vi "BRig_RT_panel_Laser2_v1,18.vi"(7 "input_setValues":bool, 9 "input_dataExp":u16[](array[numeric]), 11 "input_dataLC":u16[](array[numeric])) -> (1 "output_dataExp":u16[](array[numeric]), 3 "output_dataLC":u16[](array[numeric]))   [LabVIEW 2014]
panel:
  in  "LC_Wro_nRew2":u16
  in  "LC_Wro_nRew1":u16
  in  "LC_Rew_nRew2":u16
  in  "LC_Rew_nRew1":u16
  in  "LC_Sel_nRew2":u16
  in  "LC_Sel_nRew1":u16
  in  "LC_Cue_nRew2":u16
  in  "LC_Cue_nRew1":u16
  in  "LC_ENL_nRew2":u16
  in  "LC_ENL_nRew1":u16
  out "LaserPulseTrain":cluster{u16[], u16[]}(graph)
  in  "LED_baseline":bool
  in  "Laser_power_step":dbl
  in  "Laser_power_max":dbl
  in  "Laser_power_min":dbl
  in  "Laser_Tshutter":u16=2
  in  "Laser_Freq":u16=10
  in  "Laser_Tpeak":u16=2
  in  "Laser_T":u16
  in  "LC_Sel_PostR_Count":u16
  in  "LC_Sel_PostR_Probability":u16
  in  "LC_Sel_PostR_Block":u16(slide) max=2 step=1 scale=0.0..2.0
  in  "LC_Sel_PostR_OnOff":bool
  in  "LC_Sel_PostR_Tdelay":u16
  in  "LC_Cue_PostR_Count":u16
  in  "LC_Cue_PostR_delayOpt":bool
  in  "LC_Cue_PostR_Probability":u16
  in  "LC_Cue_PostR_Block":u16(slide) max=2 step=1 scale=0.0..2.0
  in  "LC_Cue_PostR_OnOff":bool
  in  "LC_Cue_PostR_Tdelay":u16
  in  "LC_ENL_PostR_delayOpt":bool
  in  "LC_ENL_PostR_Count":u16
  in  "LC_ENL_PostR_Probability":u16 max=100 step=1
  in  "LC_ENL_PostR_Block":u16(slide) max=2 step=1 scale=0.0..2.0
  in  "LC_ENL_PostR_OnOff":bool
  in  "LC_ENL_PostR_Tdelay":u16
  in  "LC_Sel_PreR_Count":u16
  in  "LC_Sel_First_Count":u16
  in  "LC_Sel_PreR_Probability":u16
  in  "LC_Sel_PreR_Block":u16(slide) max=2 step=1 scale=0.0..2.0
  in  "LC_Sel_PreR_OnOff":bool
  in  "LC_Sel_First_Probability":u16
  in  "LC_Sel_First_Block":u16(slide) max=2 step=1 scale=0.0..2.0
  in  "LC_Sel_First_OnOff":bool
  in  "LC_Sel_PreR_Tdelay":u16
  in  "LC_Sel_First_Tdelay":u16
  in  "LC_Cue_PreR_Count":u16
  in  "LC_Cue_First_Count":u16
  in  "LC_Cue_PreR_delayOpt":bool
  in  "LC_ENL_PreR_delayOpt":bool
  in  "LC_ENL_PreR_Count":u16
  in  "LC_ENL_First_Count":u16
  in  "LC_Cue_First_delayOpt":bool
  in  "LC_ENL_First_delayOpt":bool
  in  "LC_Wrong_Probability":u16
  in  "LC_Wrong_Trial":u16(slide) max=4 step=1 scale=0.0..4.0
  in  "LC_Wrong_Block":u16(slide) max=2 step=1 scale=0.0..2.0
  in  "LC_Wrong_OnOff":bool
  in  "LC_Reward_Probability":u16
  in  "LC_Reward_Trial":u16(slide) max=3 step=1 scale=0.0..3.0
  in  "LC_Reward_Block":u16(slide) max=2 step=1 scale=0.0..2.0
  in  "LC_Reward_OnOff":bool
  in  "LC_Cue_PreR_Probability":u16
  in  "LC_Cue_PreR_Block":u16(slide) max=2 step=1 scale=0.0..2.0
  in  "LC_Cue_PreR_OnOff":bool
  in  "LC_Cue_First_Probability":u16
  in  "LC_Cue_First_Block":u16(slide) max=2 step=1 scale=0.0..2.0
  in  "LC_Cue_First_OnOff":bool
  in  "LC_ENL_PreR_Probability":u16 max=100 step=1
  in  "LC_ENL_PreR_Block":u16(slide) max=2 step=1 scale=0.0..2.0
  in  "LC_ENL_PreR_OnOff":bool
  in  "LC_ENL_First_Probability":u16 max=100 step=1
  in  "LC_ENL_First_Block":u16(slide) max=2 step=1 scale=0.0..2.0
  in  "LC_Wrong_Tdelay":u16
  in  "LC_Cue_PreR_Tdelay":u16
  in  "LC_ENL_PreR_Tdelay":u16
  in  "LC_Reward_Tdelay":u16
  in  "LC_Cue_First_Tdelay":u16
  in  "LC_ENL_First_Tdelay":u16
  in  "LC_ENL_First_OnOff":bool
  # "Laser2 Control\n                               On/Off      Block        Probability [%]   Delay [ms]                              Count"
  # "Enforced\nNonLick"
  # "from end"
  # "First\nTrial"
  # "from start"
  # "from end"
  # "PreReward\nTrials"
  # "from start"
  # "from end"
  # "PostReward\nTrials"
  # "from start"
  # "PostReward Option - Trigger after [X1] or [X2] reward\n                                        (0 = ignore this option)"
  # "Cue"
  # "from end"
  # "First\nTrial"
  # "from start"
  # "from end"
  # "PreReward\nTrials"
  # "from start"
  # "from end"
  # "PostReward\nTrials"
  # "from start"
  # "PostReward Option - Trigger after [X1] or [X2] reward\n                                        (0 = ignore this option)"
  # "Selection"
  # "from start"
  # "First\nTrial"
  # "from start"
  # "PreReward\nTrials"
  # "from start"
  # "PostReward\nTrials"
  # "PostReward Option - Trigger after [X1] or [X2] reward\n                                        (0 = ignore this option)"
  # "Laser2 Parameters"
  # "Laser2 Response\n           On/Off      Block           Trial     Probability %  Delay [ms]"
  # "Frequency\n[Hz]"
  # "Selection\nReward"
  # "Timing [ms]\n Duration     Peak Width   Shutter"
  # "Trigger after [X1] or [X2] reward\n(0 = ignore this option)"
  # "Laser Power [V]\nMin          Max              Step"
  # "Selection\nWrong"
  # "Trigger after [X1] or [X2] reward\n(0 = ignore this option)"
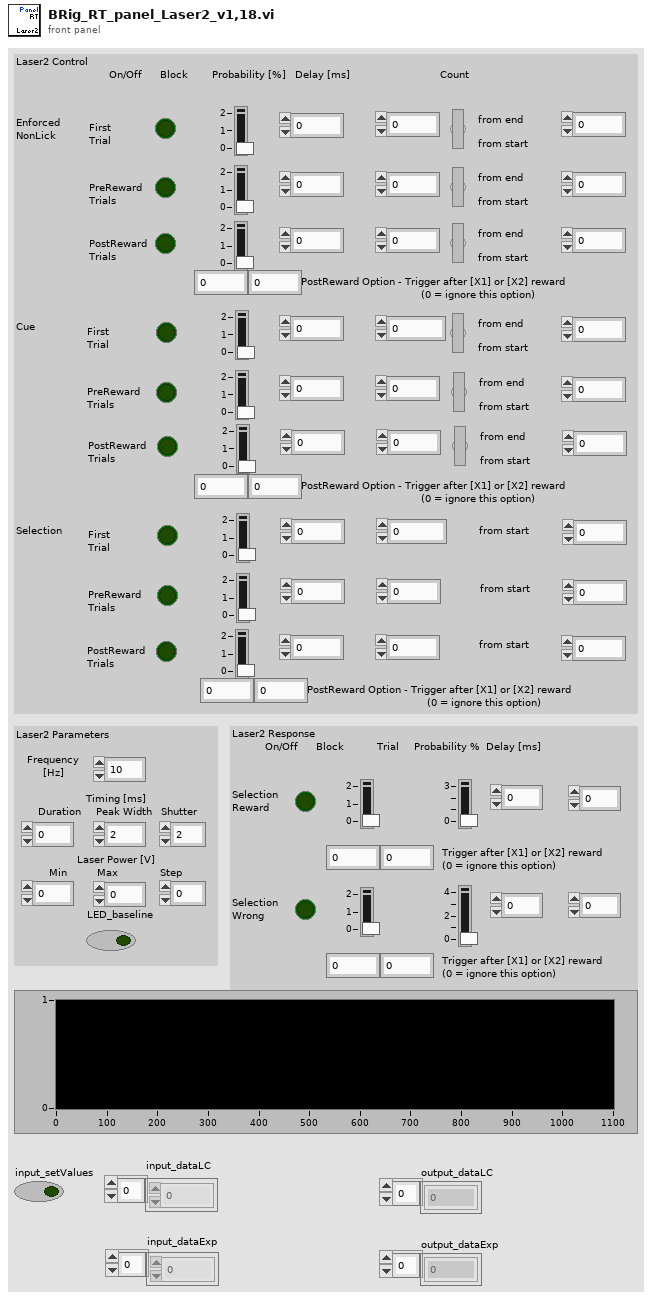
[diagram p1: front panel]
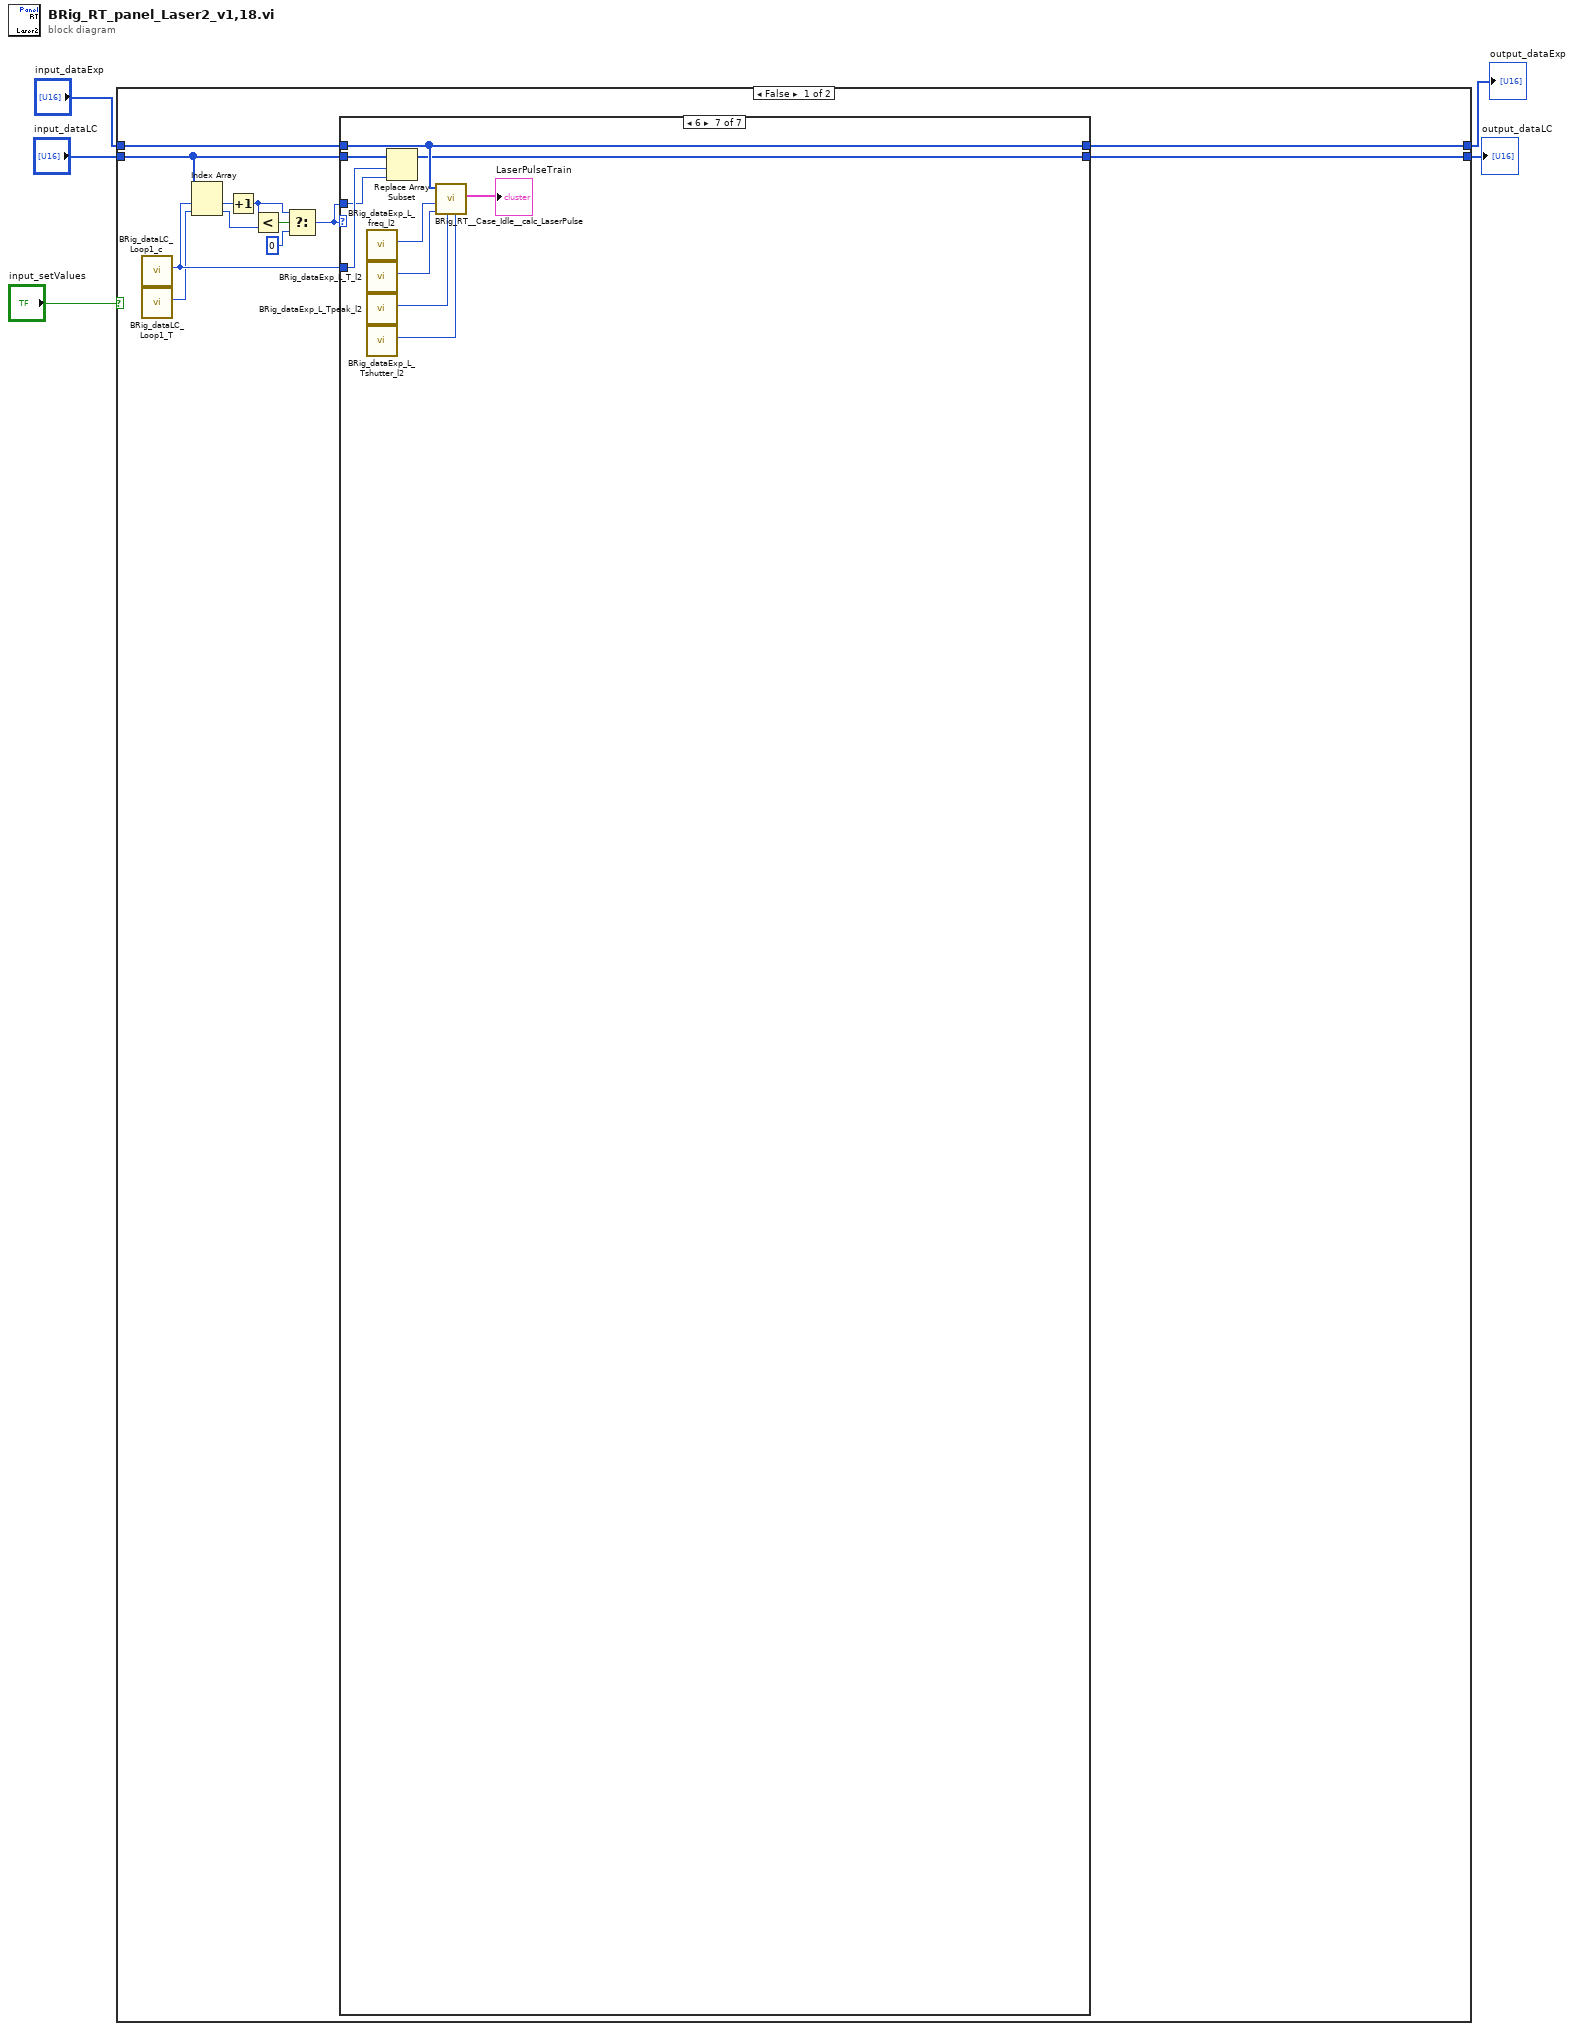
[diagram p0: block diagram]
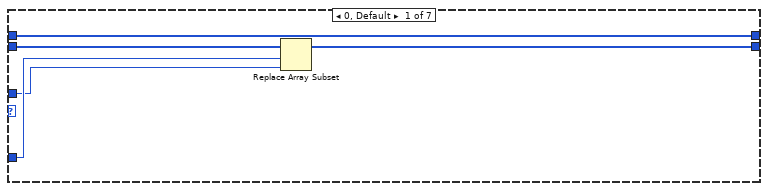
[diagram p2: hidden frame]
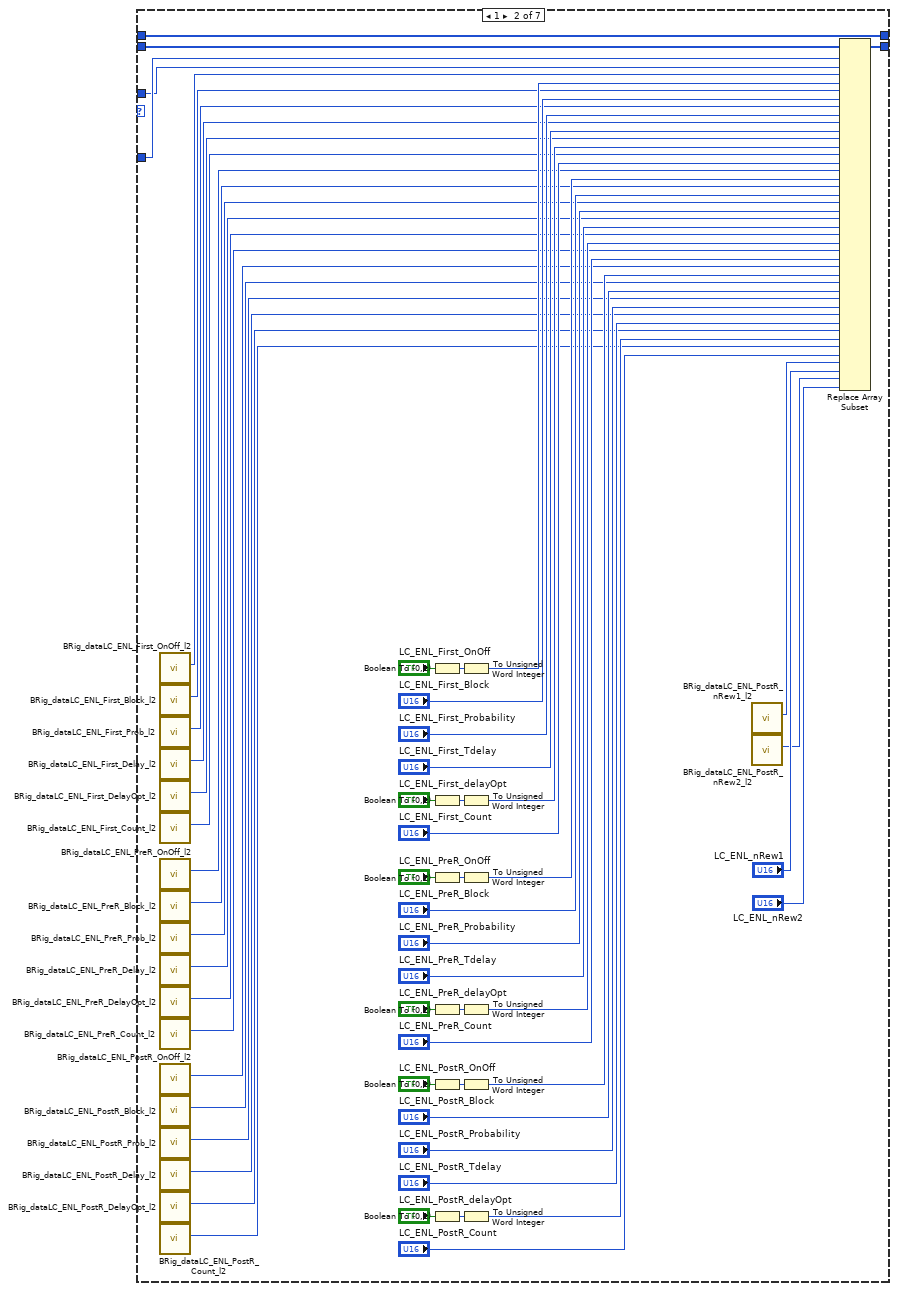
[diagram p3: hidden frame]
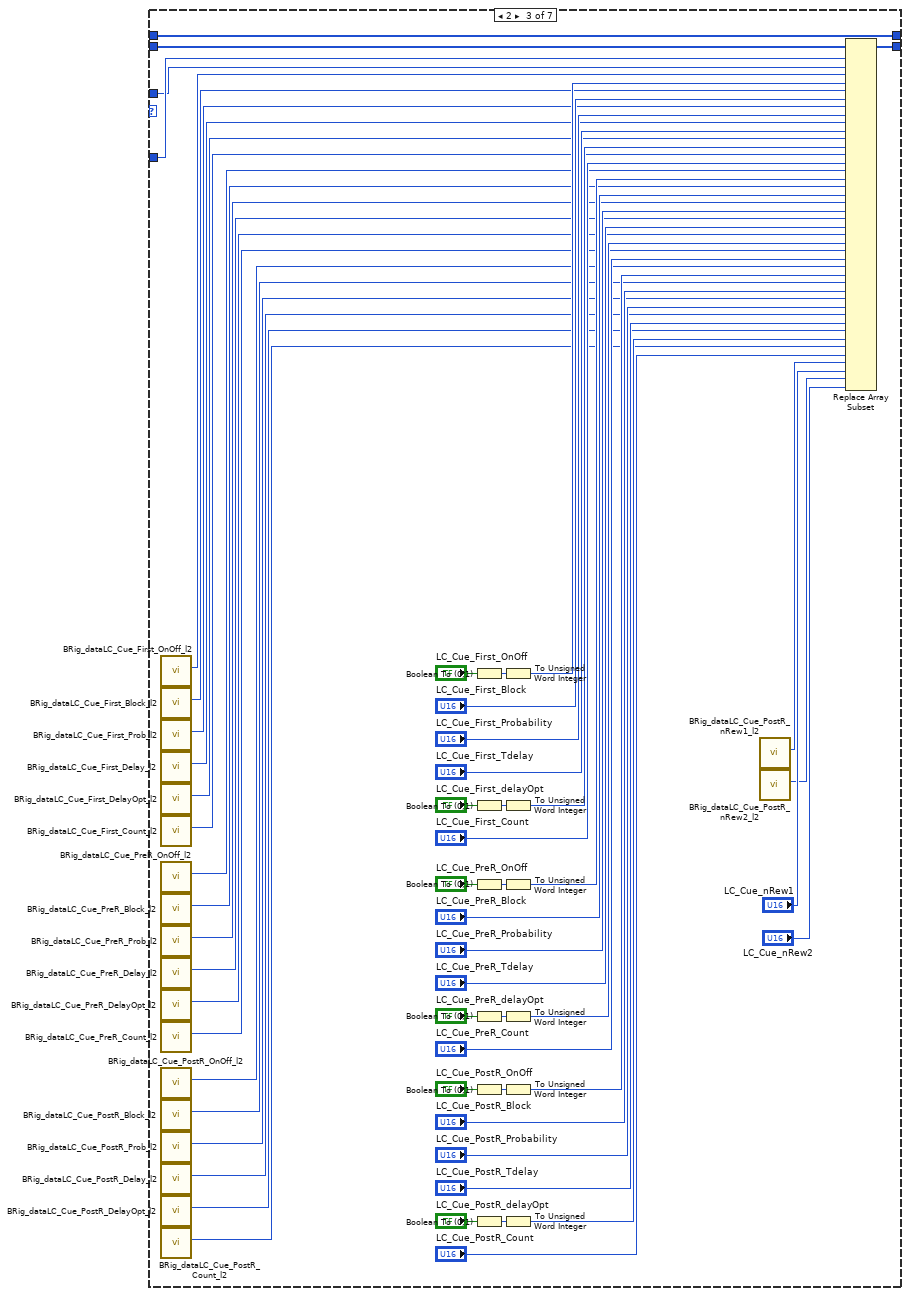
[diagram p4: hidden frame]
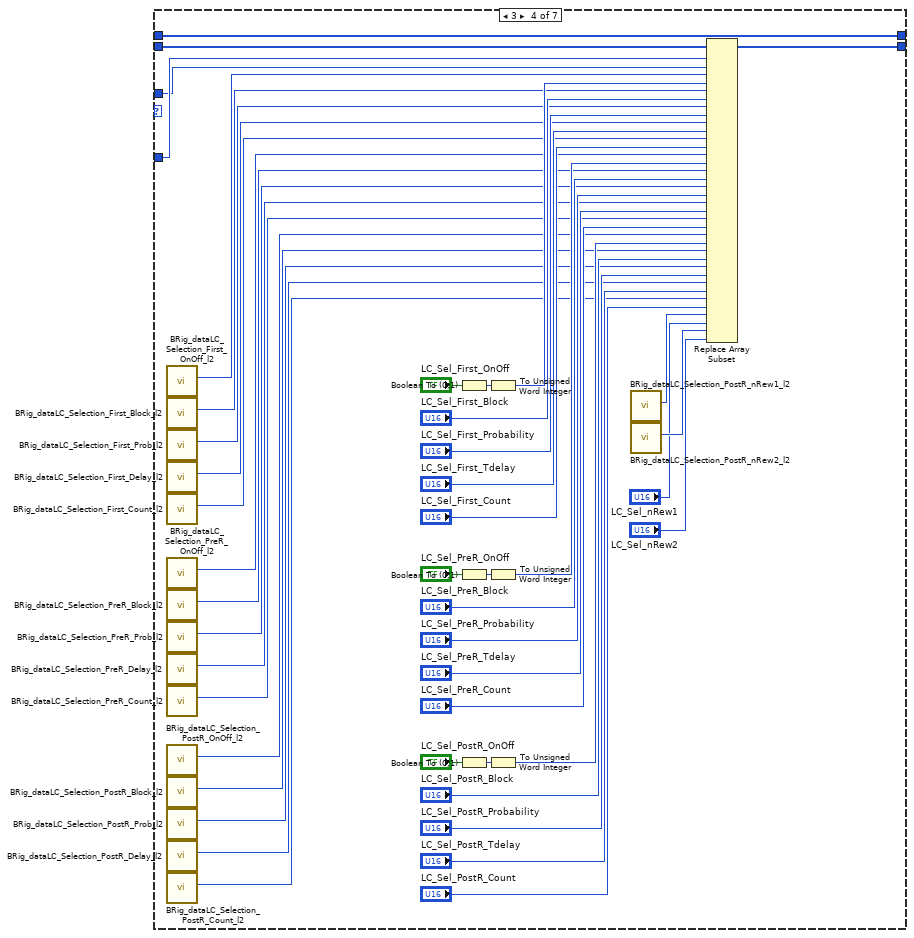
[diagram p5: hidden frame]
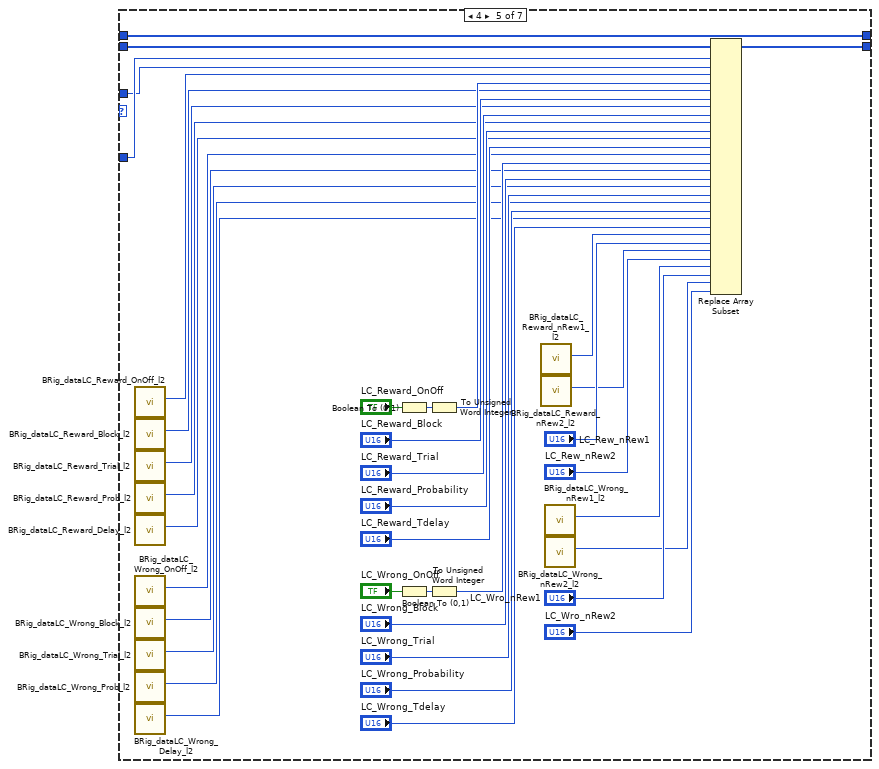
[diagram p6: hidden frame]
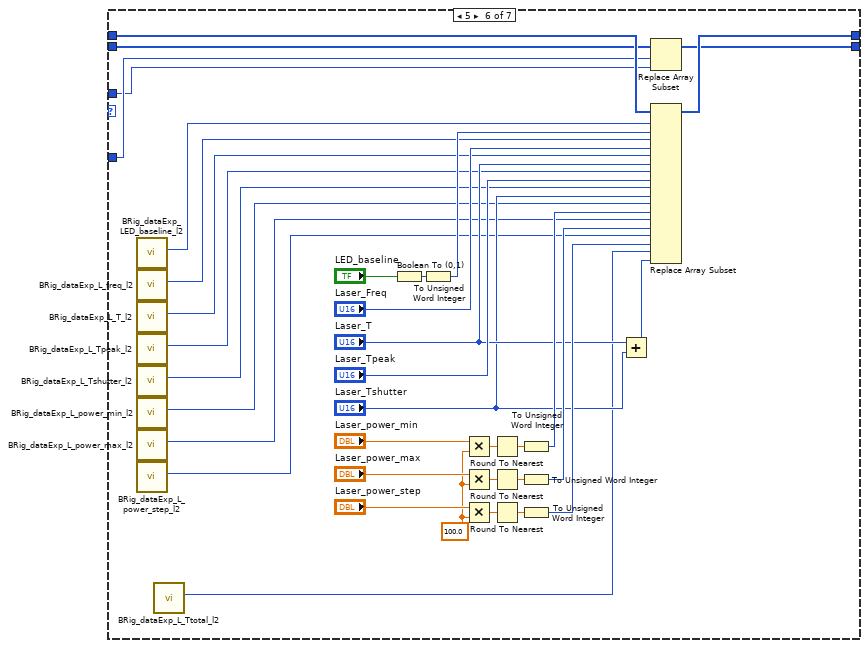
[diagram p7: hidden frame]
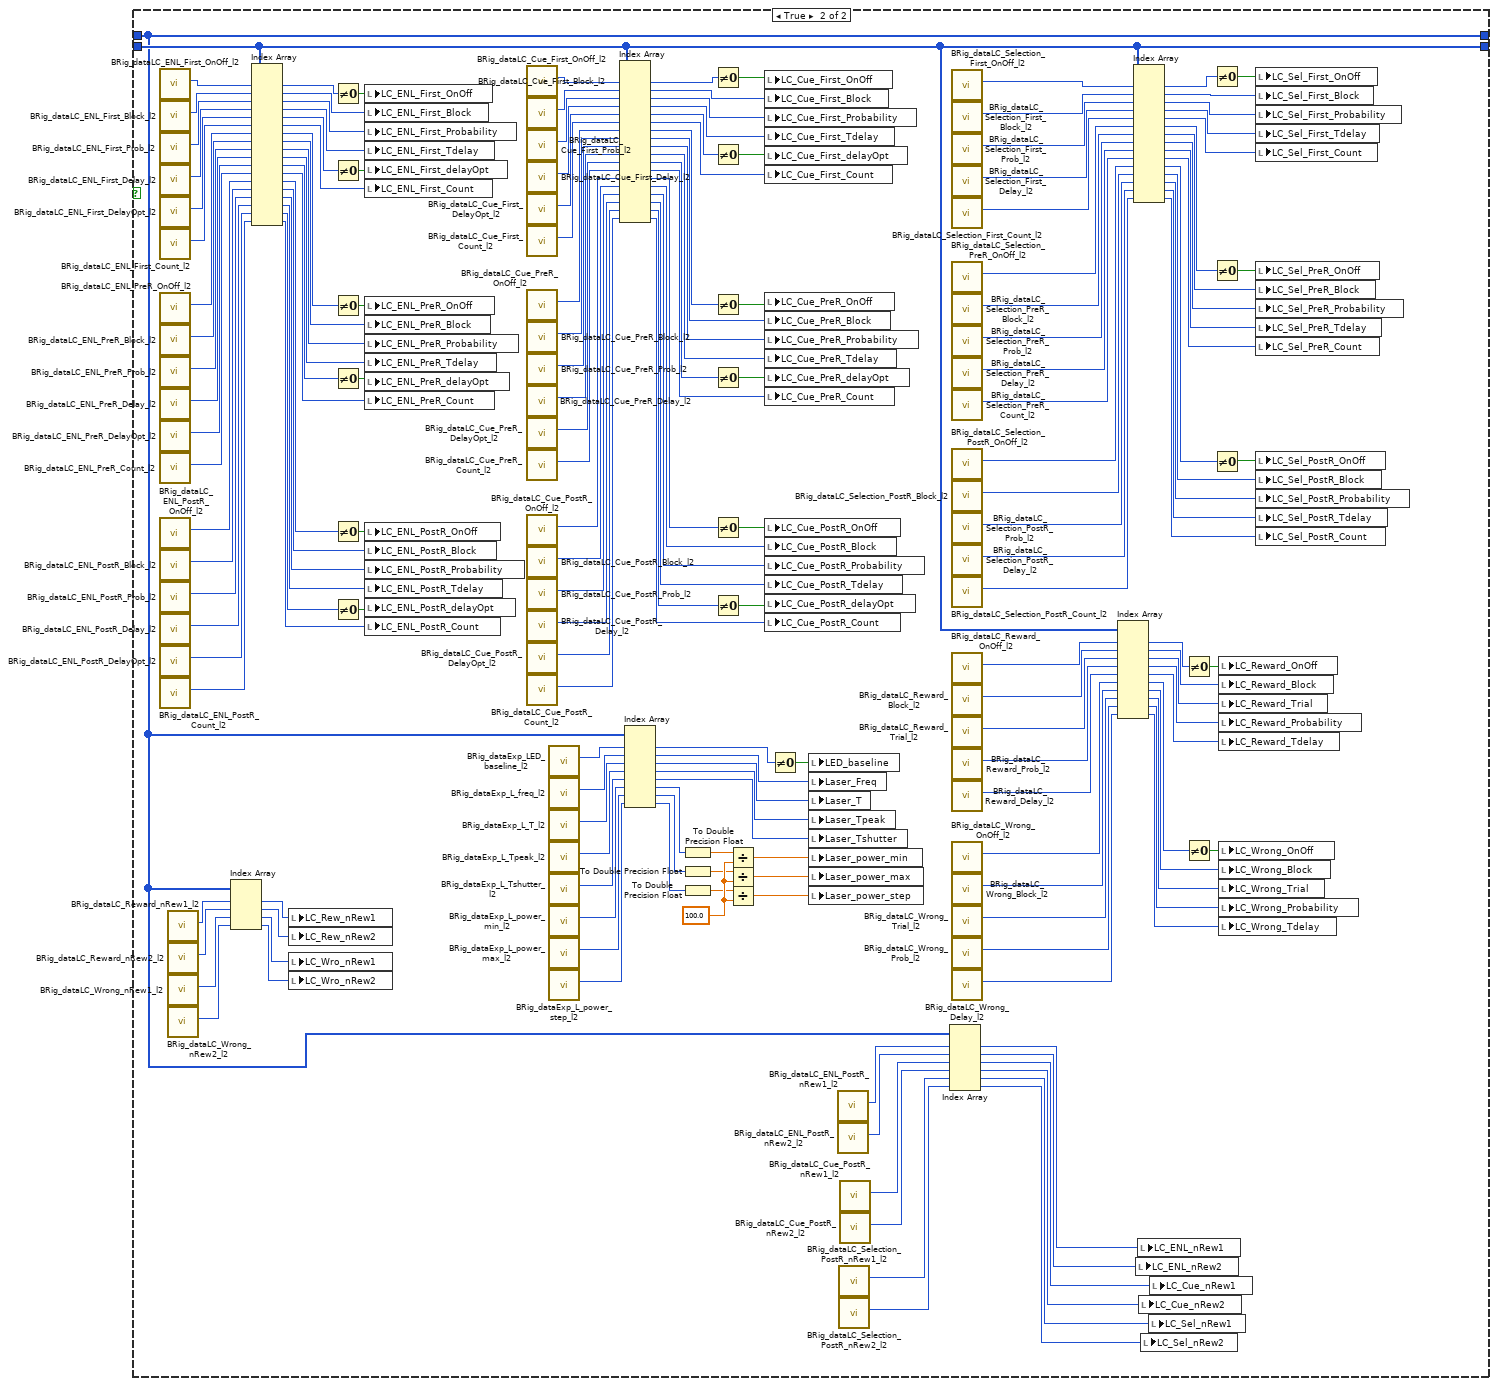
[diagram p8: hidden frame]
diagram:
  n1 = case shown="False" "input_setValues" {
    tunnel: "input_dataLC" -> [w17 w371]
    tunnel: [w11 w371] -> w4
    tunnel: "input_dataExp" -> [w7 w281]
    tunnel: [w6 w281] -> w1
    frame False {
      n2 = call "BRig_dataLC_Loop1_c.vi"() -> ("output_Loop1_c"=w10:i32)  [unwired: 11 in]
      n3 = call "BRig_dataLC_Loop1_T.vi"() -> ("output_Loop1_T"=w9:i32)  [unwired: 11 in]
      n4 = Index Array(array=w17, index #1=w10, index #2=w9) -> (element #1=w16:u16, element #2=w15:u16)
      n5 = Increment(x=w16) -> (x+1=w12:u16)
      n6 = Less?(x=w12, y=w15) -> (x < y?=w14:bool)
      n7 = Select(t=w12, s=w14, f=u16 0) -> (s? t:f=w8:u16)
      n8 = case shown="6" w8 {
        tunnel: w17 -> [w22 w79 w136 w181 w218 w231 w262]
        tunnel: w10 -> [w20 w47 w104 w158 w202 w229 w260]
        tunnel: w8 -> [w19 w46 w103 w157 w201 w228 w259]
        tunnel: [w21 w78 w135 w180 w217 w230 w261] -> w11
        tunnel: w7 -> [w18 w45 w102 w156 w200 w233 w264]
        tunnel: [w18 w45 w102 w156 w200 w232 w264] -> w6
        frame 0, Default {
          n9 = Replace Array Subset(array=w22, new element=w19, index=w20) -> (w21:u16[])
        }
        frame 1 {
          n10 = call "BRig_dataLC_ENL_First_OnOff_l2.vi"() -> ("output_ENL_First_OnOff_l2"=w27:i32)  [unwired: 11 in]
          n11 = call "BRig_dataLC_ENL_First_Block_l2.vi"() -> ("output_ENL_First_Block_l2"=w28:i32)  [unwired: 11 in]
          n12 = call "BRig_dataLC_ENL_First_Prob_l2.vi"() -> ("output_ENL_First_Prob_l2"=w29:i32)  [unwired: 11 in]
          n13 = call "BRig_dataLC_ENL_First_Delay_l2.vi"() -> ("output_ENL_First_Delay_l2"=w30:i32)  [unwired: 11 in]
          n14 = call "BRig_dataLC_ENL_First_DelayOpt_l2.vi"() -> ("output_ENL_First_DelayOpt_l2"=w31:i32)  [unwired: 11 in]
          n15 = call "BRig_dataLC_ENL_First_Count_l2.vi"() -> ("output_ENL_First_Count_l2"=w32:i32)  [unwired: 11 in]
          n16 = call "BRig_dataLC_ENL_PreR_OnOff_l2.vi"() -> ("output_ENL_PreR_OnOff_l2"=w33:i32)  [unwired: 11 in]
          n17 = call "BRig_dataLC_ENL_PreR_Block_l2.vi"() -> ("output_ENL_PreR_Block_l2"=w34:i32)  [unwired: 11 in]
          n18 = call "BRig_dataLC_ENL_PreR_Prob_l2.vi"() -> ("output_ENL_PreR_Prob_l2"=w35:i32)  [unwired: 11 in]
          n19 = call "BRig_dataLC_ENL_PreR_Delay_l2.vi"() -> ("output_ENL_PreR_Delay_l2"=w36:i32)  [unwired: 11 in]
          n20 = call "BRig_dataLC_ENL_PreR_DelayOpt_l2.vi"() -> ("output_ENL_PreR_DelayOpt_l2"=w37:i32)  [unwired: 11 in]
          n21 = call "BRig_dataLC_ENL_PreR_Count_l2.vi"() -> ("output_ENL_PreR_Count_l2"=w38:i32)  [unwired: 11 in]
          n22 = call "BRig_dataLC_ENL_PostR_OnOff_l2.vi"() -> ("output_ENL_PostR_OnOff_l2"=w39:i32)  [unwired: 11 in]
          n23 = call "BRig_dataLC_ENL_PostR_Block_l2.vi"() -> ("output_ENL_PostR_Block_l2"=w40:i32)  [unwired: 11 in]
          n24 = call "BRig_dataLC_ENL_PostR_Prob_l2.vi"() -> ("output_ENL_PostR_Prob_l2"=w41:i32)  [unwired: 11 in]
          n25 = call "BRig_dataLC_ENL_PostR_Delay_l2.vi"() -> ("output_ENL_PostR_Delay_l2"=w42:i32)  [unwired: 11 in]
          n26 = call "BRig_dataLC_ENL_PostR_DelayOpt_l2.vi"() -> ("output_ENL_PostR_DelayOpt_l2"=w43:i32)  [unwired: 11 in]
          n27 = call "BRig_dataLC_ENL_PostR_Count_l2.vi"() -> ("output_ENL_PostR_Count_l2"=w44:i32)  [unwired: 11 in]
          n28 = Boolean To (0,1)(Boolean="LC_ENL_First_OnOff") -> (0, 1=w76:i16)
          n29 = Boolean To (0,1)(Boolean="LC_ENL_First_delayOpt") -> (0, 1=w75:i16)
          n30 = Boolean To (0,1)(Boolean="LC_ENL_PreR_OnOff") -> (0, 1=w73:i16)
          n31 = Boolean To (0,1)(Boolean="LC_ENL_PreR_delayOpt") -> (0, 1=w71:i16)
          n32 = Boolean To (0,1)(Boolean="LC_ENL_PostR_OnOff") -> (0, 1=w69:i16)
          n33 = Boolean To (0,1)(Boolean="LC_ENL_PostR_delayOpt") -> (0, 1=w67:i16)
          n34 = To Unsigned Word Integer(number=w76) -> (unsigned 16bit integer=w65:u16)
          n35 = To Unsigned Word Integer(number=w75) -> (unsigned 16bit integer=w61:u16)
          n36 = To Unsigned Word Integer(number=w73) -> (unsigned 16bit integer=w59:u16)
          n37 = To Unsigned Word Integer(number=w71) -> (unsigned 16bit integer=w55:u16)
          n38 = To Unsigned Word Integer(number=w69) -> (unsigned 16bit integer=w53:u16)
          n39 = To Unsigned Word Integer(number=w67) -> (unsigned 16bit integer=w49:u16)
          n40 = call "BRig_dataLC_ENL_PostR_nRew1_l2.vi"() -> ("output_ENL_PostR_nRew1_l2"=w26:i32)  [unwired: 11 in]
          n41 = call "BRig_dataLC_ENL_PostR_nRew2_l2.vi"() -> ("output_ENL_PostR_nRew2_l2"=w24:i32)  [unwired: 11 in]
          n42 = Replace Array Subset(array=w79, new element #1=w46, index #1=w47, new element #2=w65, index #2=w27, new element #3="LC_ENL_First_Block", index #3=w28, new element #4="LC_ENL_First_Probability", index #4=w29, new element #5="LC_ENL_First_Tdelay", index #5=w30, new element #6=w61, index #6=w31, new element #7="LC_ENL_First_Count", index #7=w32, new element #8=w59, index #8=w33, new element #9="LC_ENL_PreR_Block", index #9=w34, new element #10="LC_ENL_PreR_Probability", index #10=w35, new element #11="LC_ENL_PreR_Tdelay", index #11=w36, new element #12=w55, index #12=w37, new element #13="LC_ENL_PreR_Count", index #13=w38, new element #14=w53, index #14=w39, new element #15="LC_ENL_PostR_Block", index #15=w40, new element #16="LC_ENL_PostR_Probability", index #16=w41, new element #17="LC_ENL_PostR_Tdelay", index #17=w42, new element #18=w49, index #18=w43, new element #19="LC_ENL_PostR_Count", index #19=w44, new element #20="LC_ENL_nRew1", index #20=w26, new element #21="LC_ENL_nRew2", index #21=w24) -> (w78:u16[])
        }
        frame 2 {
          n43 = call "BRig_dataLC_Cue_First_OnOff_l2.vi"() -> ("output_Cue_First_OnOff_l2"=w84:i32)  [unwired: 11 in]
          n44 = call "BRig_dataLC_Cue_First_Block_l2.vi"() -> ("output_Cue_First_Block_l2"=w85:i32)  [unwired: 11 in]
          n45 = call "BRig_dataLC_Cue_First_Prob_l2.vi"() -> ("output_Cue_First_Prob_l2"=w86:i32)  [unwired: 11 in]
          n46 = call "BRig_dataLC_Cue_First_Delay_l2.vi"() -> ("output_Cue_First_Delay_l2"=w87:i32)  [unwired: 11 in]
          n47 = call "BRig_dataLC_Cue_First_DelayOpt_l2.vi"() -> ("output_Cue_First_DelayOpt_l2"=w88:i32)  [unwired: 11 in]
          n48 = call "BRig_dataLC_Cue_First_Count_l2.vi"() -> ("output_Cue_First_Count_l2"=w89:i32)  [unwired: 11 in]
          n49 = call "BRig_dataLC_Cue_PreR_OnOff_l2.vi"() -> ("output_Cue_PreR_OnOff_l2"=w90:i32)  [unwired: 11 in]
          n50 = call "BRig_dataLC_Cue_PreR_Block_l2.vi"() -> ("output_Cue_PreR_Block_l2"=w91:i32)  [unwired: 11 in]
          n51 = call "BRig_dataLC_Cue_PreR_Prob_l2.vi"() -> ("output_Cue_PreR_Prob_l2"=w92:i32)  [unwired: 11 in]
          n52 = call "BRig_dataLC_Cue_PreR_Delay_l2.vi"() -> ("output_Cue_PreR_Delay_l2"=w93:i32)  [unwired: 11 in]
          n53 = call "BRig_dataLC_Cue_PreR_DelayOpt_l2.vi"() -> ("output_Cue_PreR_DelayOpt_l2"=w94:i32)  [unwired: 11 in]
          n54 = call "BRig_dataLC_Cue_PreR_Count_l2.vi"() -> ("output_Cue_PreR_Count_l2"=w95:i32)  [unwired: 11 in]
          n55 = call "BRig_dataLC_Cue_PostR_OnOff_l2.vi"() -> ("output_Cue_PostR_OnOff_l2"=w96:i32)  [unwired: 11 in]
          n56 = call "BRig_dataLC_Cue_PostR_Block_l2.vi"() -> ("output_Cue_PostR_Block_l2"=w97:i32)  [unwired: 11 in]
          n57 = call "BRig_dataLC_Cue_PostR_Prob_l2.vi"() -> ("output_Cue_PostR_Prob_l2"=w98:i32)  [unwired: 11 in]
          n58 = call "BRig_dataLC_Cue_PostR_Delay_l2.vi"() -> ("output_Cue_PostR_Delay_l2"=w99:i32)  [unwired: 11 in]
          n59 = call "BRig_dataLC_Cue_PostR_DelayOpt_l2.vi"() -> ("output_Cue_PostR_DelayOpt_l2"=w100:i32)  [unwired: 11 in]
          n60 = call "BRig_dataLC_Cue_PostR_Count_l2.vi"() -> ("output_Cue_PostR_Count_l2"=w101:i32)  [unwired: 11 in]
          n61 = Boolean To (0,1)(Boolean="LC_Cue_First_OnOff") -> (0, 1=w128:i16)
          n62 = Boolean To (0,1)(Boolean="LC_Cue_First_delayOpt") -> (0, 1=w127:i16)
          n63 = Boolean To (0,1)(Boolean="LC_Cue_PreR_OnOff") -> (0, 1=w126:i16)
          n64 = Boolean To (0,1)(Boolean="LC_Cue_PreR_delayOpt") -> (0, 1=w125:i16)
          n65 = Boolean To (0,1)(Boolean="LC_Cue_PostR_OnOff") -> (0, 1=w124:i16)
          n66 = Boolean To (0,1)(Boolean="LC_Cue_PostR_delayOpt") -> (0, 1=w123:i16)
          n67 = To Unsigned Word Integer(number=w128) -> (unsigned 16bit integer=w122:u16)
          n68 = To Unsigned Word Integer(number=w127) -> (unsigned 16bit integer=w118:u16)
          n69 = To Unsigned Word Integer(number=w126) -> (unsigned 16bit integer=w116:u16)
          n70 = To Unsigned Word Integer(number=w125) -> (unsigned 16bit integer=w112:u16)
          n71 = To Unsigned Word Integer(number=w124) -> (unsigned 16bit integer=w110:u16)
          n72 = To Unsigned Word Integer(number=w123) -> (unsigned 16bit integer=w106:u16)
          n73 = call "BRig_dataLC_Cue_PostR_nRew1_l2.vi"() -> ("output_Cue_PostR_nRew1_l2"=w83:i32)  [unwired: 11 in]
          n74 = call "BRig_dataLC_Cue_PostR_nRew2_l2.vi"() -> ("output_Cue_PostR_nRew2_l2"=w81:i32)  [unwired: 11 in]
          n75 = Replace Array Subset(array=w136, new element #1=w103, index #1=w104, new element #2=w122, index #2=w84, new element #3="LC_Cue_First_Block", index #3=w85, new element #4="LC_Cue_First_Probability", index #4=w86, new element #5="LC_Cue_First_Tdelay", index #5=w87, new element #6=w118, index #6=w88, new element #7="LC_Cue_First_Count", index #7=w89, new element #8=w116, index #8=w90, new element #9="LC_Cue_PreR_Block", index #9=w91, new element #10="LC_Cue_PreR_Probability", index #10=w92, new element #11="LC_Cue_PreR_Tdelay", index #11=w93, new element #12=w112, index #12=w94, new element #13="LC_Cue_PreR_Count", index #13=w95, new element #14=w110, index #14=w96, new element #15="LC_Cue_PostR_Block", index #15=w97, new element #16="LC_Cue_PostR_Probability", index #16=w98, new element #17="LC_Cue_PostR_Tdelay", index #17=w99, new element #18=w106, index #18=w100, new element #19="LC_Cue_PostR_Count", index #19=w101, new element #20="LC_Cue_nRew1", index #20=w83, new element #21="LC_Cue_nRew2", index #21=w81) -> (w135:u16[])
        }
        frame 3 {
          n76 = call "BRig_dataLC_Selection_First_OnOff_l2.vi"() -> ("output_Selection_First_OnOff_l2"=w141:i32)  [unwired: 11 in]
          n77 = call "BRig_dataLC_Selection_First_Block_l2.vi"() -> ("output_Selection_First_Block_l2"=w142:i32)  [unwired: 11 in]
          n78 = call "BRig_dataLC_Selection_First_Prob_l2.vi"() -> ("output_Selection_First_Prob_l2"=w143:i32)  [unwired: 11 in]
          n79 = call "BRig_dataLC_Selection_First_Delay_l2.vi"() -> ("output_Selection_First_Delay_l2"=w144:i32)  [unwired: 11 in]
          n80 = call "BRig_dataLC_Selection_First_Count_l2.vi"() -> ("output_Selection_First_Count_l2"=w145:i32)  [unwired: 11 in]
          n81 = call "BRig_dataLC_Selection_PreR_OnOff_l2.vi"() -> ("output_Selection_PreR_OnOff_l2"=w146:i32)  [unwired: 11 in]
          n82 = call "BRig_dataLC_Selection_PreR_Block_l2.vi"() -> ("output_Selection_PreR_Block_l2"=w147:i32)  [unwired: 11 in]
          n83 = call "BRig_dataLC_Selection_PreR_Prob_l2.vi"() -> ("output_Selection_PreR_Prob_l2"=w148:i32)  [unwired: 11 in]
          n84 = call "BRig_dataLC_Selection_PreR_Delay_l2.vi"() -> ("output_Selection_PreR_Delay_l2"=w149:i32)  [unwired: 11 in]
          n85 = call "BRig_dataLC_Selection_PreR_Count_l2.vi"() -> ("output_Selection_PreR_Count_l2"=w150:i32)  [unwired: 11 in]
          n86 = call "BRig_dataLC_Selection_PostR_OnOff_l2.vi"() -> ("output_Selection_PostR_OnOff_l2"=w151:i32)  [unwired: 11 in]
          n87 = call "BRig_dataLC_Selection_PostR_Block_l2.vi"() -> ("output_Selection_PostR_Block_l2"=w152:i32)  [unwired: 11 in]
          n88 = call "BRig_dataLC_Selection_PostR_Prob_l2.vi"() -> ("output_Selection_PostR_Prob_l2"=w153:i32)  [unwired: 11 in]
          n89 = call "BRig_dataLC_Selection_PostR_Delay_l2.vi"() -> ("output_Selection_PostR_Delay_l2"=w154:i32)  [unwired: 11 in]
          n90 = call "BRig_dataLC_Selection_PostR_Count_l2.vi"() -> ("output_Selection_PostR_Count_l2"=w155:i32)  [unwired: 11 in]
          n91 = Boolean To (0,1)(Boolean="LC_Sel_First_OnOff") -> (0, 1=w176:i16)
          n92 = Boolean To (0,1)(Boolean="LC_Sel_PreR_OnOff") -> (0, 1=w175:i16)
          n93 = Boolean To (0,1)(Boolean="LC_Sel_PostR_OnOff") -> (0, 1=w174:i16)
          n94 = To Unsigned Word Integer(number=w176) -> (unsigned 16bit integer=w173:u16)
          n95 = To Unsigned Word Integer(number=w175) -> (unsigned 16bit integer=w168:u16)
          n96 = To Unsigned Word Integer(number=w174) -> (unsigned 16bit integer=w163:u16)
          n97 = call "BRig_dataLC_Selection_PostR_nRew1_l2.vi"() -> ("output_Selection_PostR_nRew1_l2"=w140:i32)  [unwired: 11 in]
          n98 = call "BRig_dataLC_Selection_PostR_nRew2_l2.vi"() -> ("output_Selection_PostR_nRew2_l2"=w139:i32)  [unwired: 11 in]
          n99 = Replace Array Subset(array=w181, new element #1=w157, index #1=w158, new element #2=w173, index #2=w141, new element #3="LC_Sel_First_Block", index #3=w142, new element #4="LC_Sel_First_Probability", index #4=w143, new element #5="LC_Sel_First_Tdelay", index #5=w144, new element #6="LC_Sel_First_Count", index #6=w145, new element #7=w168, index #7=w146, new element #8="LC_Sel_PreR_Block", index #8=w147, new element #9="LC_Sel_PreR_Probability", index #9=w148, new element #10="LC_Sel_PreR_Tdelay", index #10=w149, new element #11="LC_Sel_PreR_Count", index #11=w150, new element #12=w163, index #12=w151, new element #13="LC_Sel_PostR_Block", index #13=w152, new element #14="LC_Sel_PostR_Probability", index #14=w153, new element #15="LC_Sel_PostR_Tdelay", index #15=w154, new element #16="LC_Sel_PostR_Count", index #16=w155, new element #17="LC_Sel_nRew1", index #17=w140, new element #18="LC_Sel_nRew2", index #18=w139) -> (w180:u16[])
        }
        frame 4 {
          n100 = call "BRig_dataLC_Reward_OnOff_l2.vi"() -> ("output_Reward_OnOff_l2"=w190:i32)  [unwired: 11 in]
          n101 = call "BRig_dataLC_Reward_Block_l2.vi"() -> ("output_Reward_Block_l2"=w191:i32)  [unwired: 11 in]
          n102 = call "BRig_dataLC_Reward_Trial_l2.vi"() -> ("output_Reward_Trial_l2"=w192:i32)  [unwired: 11 in]
          n103 = call "BRig_dataLC_Reward_Prob_l2.vi"() -> ("output_Reward_Prob_l2"=w193:i32)  [unwired: 11 in]
          n104 = call "BRig_dataLC_Reward_Delay_l2.vi"() -> ("output_Reward_Delay_l2"=w194:i32)  [unwired: 11 in]
          n105 = call "BRig_dataLC_Wrong_OnOff_l2.vi"() -> ("output_Wrong_OnOff_l2"=w195:i32)  [unwired: 11 in]
          n106 = call "BRig_dataLC_Wrong_Block_l2.vi"() -> ("output_Wrong_Block_l2"=w196:i32)  [unwired: 11 in]
          n107 = call "BRig_dataLC_Wrong_Trial_l2.vi"() -> ("output_Wrong_Trial_l2"=w197:i32)  [unwired: 11 in]
          n108 = call "BRig_dataLC_Wrong_Prob_l2.vi"() -> ("output_Wrong_Prob_l2"=w198:i32)  [unwired: 11 in]
          n109 = call "BRig_dataLC_Wrong_Delay_l2.vi"() -> ("output_Wrong_Delay_l2"=w199:i32)  [unwired: 11 in]
          n110 = Boolean To (0,1)(Boolean="LC_Reward_OnOff") -> (0, 1=w214:i16)
          n111 = Boolean To (0,1)(Boolean="LC_Wrong_OnOff") -> (0, 1=w213:i16)
          n112 = To Unsigned Word Integer(number=w214) -> (unsigned 16bit integer=w212:u16)
          n113 = To Unsigned Word Integer(number=w213) -> (unsigned 16bit integer=w207:u16)
          n114 = call "BRig_dataLC_Reward_nRew1_l2.vi"() -> ("output_Reward_nRew1_l2"=w186:i32)  [unwired: 11 in]
          n115 = call "BRig_dataLC_Reward_nRew2_l2.vi"() -> ("output_Reward_nRew2_l2"=w187:i32)  [unwired: 11 in]
          n116 = call "BRig_dataLC_Wrong_nRew1_l2.vi"() -> ("output_Wrong_nRew1_l2"=w185:i32)  [unwired: 11 in]
          n117 = call "BRig_dataLC_Wrong_nRew2_l2.vi"() -> ("output_Wrong_nRew2_l2"=w183:i32)  [unwired: 11 in]
          n118 = Replace Array Subset(array=w218, new element #1=w201, index #1=w202, new element #2=w212, index #2=w190, new element #3="LC_Reward_Block", index #3=w191, new element #4="LC_Reward_Trial", index #4=w192, new element #5="LC_Reward_Probability", index #5=w193, new element #6="LC_Reward_Tdelay", index #6=w194, new element #7=w207, index #7=w195, new element #8="LC_Wrong_Block", index #8=w196, new element #9="LC_Wrong_Trial", index #9=w197, new element #10="LC_Wrong_Probability", index #10=w198, new element #11="LC_Wrong_Tdelay", index #11=w199, new element #12="LC_Rew_nRew1", index #12=w186, new element #13="LC_Rew_nRew2", index #13=w187, new element #14="LC_Wro_nRew1", index #14=w185, new element #15="LC_Wro_nRew2", index #15=w183) -> (w217:u16[])
        }
        frame 5 {
          w242 = 100.0 ("y")
          n119 = call "BRig_dataExp_LED_baseline_l2.vi"() -> ("output_LED_baseline_l2"=w219:i32)  [unwired: 11 in]
          n120 = call "BRig_dataExp_L_freq_l2.vi"() -> ("output_L_freq_l2"=w220:i32)  [unwired: 11 in]
          n121 = call "BRig_dataExp_L_T_l2.vi"() -> ("output_L_T_l2"=w221:i32)  [unwired: 11 in]
          n122 = call "BRig_dataExp_L_Tpeak_l2.vi"() -> ("output_L_Tpeak_l2"=w222:i32)  [unwired: 11 in]
          n123 = call "BRig_dataExp_L_Tshutter_l2.vi"() -> ("output_L_Tshutter_l2"=w223:i32)  [unwired: 11 in]
          n124 = call "BRig_dataExp_L_power_min_l2.vi"() -> ("output_L_power_min_l2"=w224:i32)  [unwired: 11 in]
          n125 = call "BRig_dataExp_L_power_max_l2.vi"() -> ("output_L_power_max_l2"=w225:i32)  [unwired: 11 in]
          n126 = call "BRig_dataExp_L_power_step_l2.vi"() -> ("output_L_power_step_l2"=w226:i32)  [unwired: 11 in]
          n127 = call "BRig_dataExp_L_Ttotal_l2.vi"() -> ("output_L_Ttotal_l2"=w227:i32)  [unwired: 11 in]
          n128 = Boolean To (0,1)(Boolean="LED_baseline") -> (0, 1=w254:i16)
          n129 = To Unsigned Word Integer(number=w254) -> (unsigned 16bit integer=w252:u16)
          n130 = Multiply(x="Laser_power_min", y=w242) -> (x*y=w246:dbl)
          n131 = Multiply(x="Laser_power_max", y=w242) -> (x*y=w248:dbl)
          n132 = Multiply(x="Laser_power_step", y=w242) -> (x*y=w251:dbl)
          n133 = Round To Nearest(number=w246) -> (nearest integer value=w245:dbl)
          n134 = Round To Nearest(number=w248) -> (nearest integer value=w247:dbl)
          n135 = Round To Nearest(number=w251) -> (nearest integer value=w250:dbl)
          n136 = To Unsigned Word Integer(number=w245) -> (unsigned 16bit integer=w239:u16)
          n137 = To Unsigned Word Integer(number=w247) -> (unsigned 16bit integer=w240:u16)
          n138 = To Unsigned Word Integer(number=w250) -> (unsigned 16bit integer=w241:u16)
          n139 = Add(x="Laser_T", y="Laser_Tshutter") -> (x+y=w234:u16)
          n140 = Replace Array Subset(array=w231, new element=w228, index=w229) -> (w230:u16[])
          n141 = Replace Array Subset(array=w233, new element #1=w252, index #1=w219, new element #2="Laser_Freq", index #2=w220, new element #3="Laser_T", index #3=w221, new element #4="Laser_Tpeak", index #4=w222, new element #5="Laser_Tshutter", index #5=w223, new element #6=w239, index #6=w224, new element #7=w240, index #7=w225, new element #8=w241, index #8=w226, new element #9=w234, index #9=w227) -> (w232:u16[])
        }
        frame 6 {
          n142 = call "BRig_dataExp_L_freq_l2.vi"() -> ("output_L_freq_l2"=w255:i32)  [unwired: 11 in]
          n143 = call "BRig_dataExp_L_T_l2.vi"() -> ("output_L_T_l2"=w256:i32)  [unwired: 11 in]
          n144 = call "BRig_dataExp_L_Tpeak_l2.vi"() -> ("output_L_Tpeak_l2"=w257:i32)  [unwired: 11 in]
          n145 = call "BRig_dataExp_L_Tshutter_l2.vi"() -> ("output_L_Tshutter_l2"=w258:i32)  [unwired: 11 in]
          n146 = Replace Array Subset(array=w262, new element=w259, index=w260) -> (w261:u16[])
          n147 = call "BRig_RT__Case_Idle__calc_LaserPulse.vi"("input_dataExp_L_Tshutter"=w258, "input_dataExp_L_Tpeak"=w257, "input_dataExp_L_T"=w256, "input_dataExp_L_freq"=w255, "input_dataExp"=w264) -> ("output_cluster"=→"LaserPulseTrain":cluster{u16[], u16[]})  [unwired: 6 in]
        }
      }
    }
    frame True {
      w357 = 100.0 ("y")
      n148 = call "BRig_dataLC_ENL_First_OnOff_l2.vi"() -> ("output_ENL_First_OnOff_l2"=w334:i32)  [unwired: 11 in]
      n149 = call "BRig_dataLC_ENL_First_Block_l2.vi"() -> ("output_ENL_First_Block_l2"=w333:i32)  [unwired: 11 in]
      n150 = call "BRig_dataLC_ENL_First_Prob_l2.vi"() -> ("output_ENL_First_Prob_l2"=w335:i32)  [unwired: 11 in]
      n151 = call "BRig_dataLC_ENL_First_Delay_l2.vi"() -> ("output_ENL_First_Delay_l2"=w336:i32)  [unwired: 11 in]
      n152 = call "BRig_dataLC_ENL_First_DelayOpt_l2.vi"() -> ("output_ENL_First_DelayOpt_l2"=w337:i32)  [unwired: 11 in]
      n153 = call "BRig_dataLC_ENL_First_Count_l2.vi"() -> ("output_ENL_First_Count_l2"=w338:i32)  [unwired: 11 in]
      n154 = call "BRig_dataLC_ENL_PreR_OnOff_l2.vi"() -> ("output_ENL_PreR_OnOff_l2"=w339:i32)  [unwired: 11 in]
      n155 = call "BRig_dataLC_ENL_PreR_Block_l2.vi"() -> ("output_ENL_PreR_Block_l2"=w340:i32)  [unwired: 11 in]
      n156 = call "BRig_dataLC_ENL_PreR_Prob_l2.vi"() -> ("output_ENL_PreR_Prob_l2"=w341:i32)  [unwired: 11 in]
      n157 = call "BRig_dataLC_ENL_PreR_Delay_l2.vi"() -> ("output_ENL_PreR_Delay_l2"=w342:i32)  [unwired: 11 in]
      n158 = call "BRig_dataLC_ENL_PreR_DelayOpt_l2.vi"() -> ("output_ENL_PreR_DelayOpt_l2"=w343:i32)  [unwired: 11 in]
      n159 = call "BRig_dataLC_ENL_PreR_Count_l2.vi"() -> ("output_ENL_PreR_Count_l2"=w344:i32)  [unwired: 11 in]
      n160 = call "BRig_dataLC_ENL_PostR_OnOff_l2.vi"() -> ("output_ENL_PostR_OnOff_l2"=w345:i32)  [unwired: 11 in]
      n161 = call "BRig_dataLC_ENL_PostR_Block_l2.vi"() -> ("output_ENL_PostR_Block_l2"=w346:i32)  [unwired: 11 in]
      n162 = call "BRig_dataLC_ENL_PostR_Prob_l2.vi"() -> ("output_ENL_PostR_Prob_l2"=w347:i32)  [unwired: 11 in]
      n163 = call "BRig_dataLC_ENL_PostR_Delay_l2.vi"() -> ("output_ENL_PostR_Delay_l2"=w348:i32)  [unwired: 11 in]
      n164 = call "BRig_dataLC_ENL_PostR_DelayOpt_l2.vi"() -> ("output_ENL_PostR_DelayOpt_l2"=w349:i32)  [unwired: 11 in]
      n165 = call "BRig_dataLC_ENL_PostR_Count_l2.vi"() -> ("output_ENL_PostR_Count_l2"=w350:i32)  [unwired: 11 in]
      n166 = call "BRig_dataLC_Reward_nRew1_l2.vi"() -> ("output_Reward_nRew1_l2"=w280:i32)  [unwired: 11 in]
      n167 = call "BRig_dataLC_Reward_nRew2_l2.vi"() -> ("output_Reward_nRew2_l2"=w279:i32)  [unwired: 11 in]
      n168 = call "BRig_dataLC_Wrong_nRew1_l2.vi"() -> ("output_Wrong_nRew1_l2"=w276:i32)  [unwired: 11 in]
      n169 = call "BRig_dataLC_Wrong_nRew2_l2.vi"() -> ("output_Wrong_nRew2_l2"=w275:i32)  [unwired: 11 in]
      n170 = Index Array(array=w281, index #1=w280, index #2=w279, index #3=w276, index #4=w275) -> (element #1=w278:u16, element #2=w277:u16, element #3=w274:u16, element #4=w273:u16)
      n171 = Index Array(array=w371, index #1=w334, index #2=w333, index #3=w335, index #4=w336, index #5=w337, index #6=w338, index #7=w339, index #8=w340, index #9=w341, index #10=w342, index #11=w343, index #12=w344, index #13=w345, index #14=w346, index #15=w347, index #16=w348, index #17=w349, index #18=w350) -> (element #1=w443:u16, element #2=w442:u16, element #3=w441:u16, element #4=w440:u16, element #5=w439:u16, element #6=w438:u16, element #7=w437:u16, element #8=w436:u16, element #9=w435:u16, element #10=w434:u16, element #11=w433:u16, element #12=w432:u16, element #13=w431:u16, element #14=w430:u16, element #15=w429:u16, element #16=w428:u16, element #17=w427:u16, element #18=w426:u16)
      n172 = local write "LC_Rew_nRew1"(w278) -> ()
      n173 = local write "LC_Rew_nRew2"(w277) -> ()
      n174 = local write "LC_Wro_nRew1"(w274) -> ()
      n175 = local write "LC_Wro_nRew2"(w273) -> ()
      n176 = Not Equal To 0?(x=w443) -> (x != 0?=w449:bool)
      n177 = Not Equal To 0?(x=w439) -> (x != 0?=w448:bool)
      n178 = Not Equal To 0?(x=w437) -> (x != 0?=w447:bool)
      n179 = Not Equal To 0?(x=w433) -> (x != 0?=w446:bool)
      n180 = Not Equal To 0?(x=w431) -> (x != 0?=w445:bool)
      n181 = Not Equal To 0?(x=w427) -> (x != 0?=w444:bool)
      n182 = local write "LC_ENL_First_OnOff"(w449) -> ()
      n183 = local write "LC_ENL_First_Block"(w442) -> ()
      n184 = local write "LC_ENL_First_Probability"(w441) -> ()
      n185 = local write "LC_ENL_First_Tdelay"(w440) -> ()
      n186 = local write "LC_ENL_First_delayOpt"(w448) -> ()
      n187 = local write "LC_ENL_First_Count"(w438) -> ()
      n188 = local write "LC_ENL_PreR_OnOff"(w447) -> ()
      n189 = local write "LC_ENL_PreR_Block"(w436) -> ()
      n190 = local write "LC_ENL_PreR_Probability"(w435) -> ()
      n191 = local write "LC_ENL_PreR_Tdelay"(w434) -> ()
      n192 = local write "LC_ENL_PreR_delayOpt"(w446) -> ()
      n193 = local write "LC_ENL_PreR_Count"(w432) -> ()
      n194 = local write "LC_ENL_PostR_OnOff"(w445) -> ()
      n195 = local write "LC_ENL_PostR_Block"(w430) -> ()
      n196 = local write "LC_ENL_PostR_Probability"(w429) -> ()
      n197 = local write "LC_ENL_PostR_Tdelay"(w428) -> ()
      n198 = local write "LC_ENL_PostR_delayOpt"(w444) -> ()
      n199 = local write "LC_ENL_PostR_Count"(w426) -> ()
      n200 = call "BRig_dataLC_Cue_First_OnOff_l2.vi"() -> ("output_Cue_First_OnOff_l2"=w317:i32)  [unwired: 11 in]
      n201 = call "BRig_dataLC_Cue_First_Block_l2.vi"() -> ("output_Cue_First_Block_l2"=w315:i32)  [unwired: 11 in]
      n202 = call "BRig_dataLC_Cue_First_Prob_l2.vi"() -> ("output_Cue_First_Prob_l2"=w316:i32)  [unwired: 11 in]
      n203 = call "BRig_dataLC_Cue_First_Delay_l2.vi"() -> ("output_Cue_First_Delay_l2"=w318:i32)  [unwired: 11 in]
      n204 = call "BRig_dataLC_Cue_First_DelayOpt_l2.vi"() -> ("output_Cue_First_DelayOpt_l2"=w319:i32)  [unwired: 11 in]
      n205 = call "BRig_dataLC_Cue_First_Count_l2.vi"() -> ("output_Cue_First_Count_l2"=w320:i32)  [unwired: 11 in]
      n206 = call "BRig_dataLC_Cue_PreR_OnOff_l2.vi"() -> ("output_Cue_PreR_OnOff_l2"=w321:i32)  [unwired: 11 in]
      n207 = call "BRig_dataLC_Cue_PreR_Block_l2.vi"() -> ("output_Cue_PreR_Block_l2"=w322:i32)  [unwired: 11 in]
      n208 = call "BRig_dataLC_Cue_PreR_Prob_l2.vi"() -> ("output_Cue_PreR_Prob_l2"=w323:i32)  [unwired: 11 in]
      n209 = call "BRig_dataLC_Cue_PreR_Delay_l2.vi"() -> ("output_Cue_PreR_Delay_l2"=w324:i32)  [unwired: 11 in]
      n210 = call "BRig_dataLC_Cue_PreR_DelayOpt_l2.vi"() -> ("output_Cue_PreR_DelayOpt_l2"=w325:i32)  [unwired: 11 in]
      n211 = call "BRig_dataLC_Cue_PreR_Count_l2.vi"() -> ("output_Cue_PreR_Count_l2"=w326:i32)  [unwired: 11 in]
      n212 = call "BRig_dataLC_Cue_PostR_OnOff_l2.vi"() -> ("output_Cue_PostR_OnOff_l2"=w327:i32)  [unwired: 11 in]
      n213 = call "BRig_dataLC_Cue_PostR_Block_l2.vi"() -> ("output_Cue_PostR_Block_l2"=w328:i32)  [unwired: 11 in]
      n214 = call "BRig_dataLC_Cue_PostR_Prob_l2.vi"() -> ("output_Cue_PostR_Prob_l2"=w329:i32)  [unwired: 11 in]
      n215 = call "BRig_dataLC_Cue_PostR_Delay_l2.vi"() -> ("output_Cue_PostR_Delay_l2"=w330:i32)  [unwired: 11 in]
      n216 = call "BRig_dataLC_Cue_PostR_DelayOpt_l2.vi"() -> ("output_Cue_PostR_DelayOpt_l2"=w331:i32)  [unwired: 11 in]
      n217 = call "BRig_dataLC_Cue_PostR_Count_l2.vi"() -> ("output_Cue_PostR_Count_l2"=w332:i32)  [unwired: 11 in]
      n218 = call "BRig_dataExp_LED_baseline_l2.vi"() -> ("output_LED_baseline_l2"=w289:i32)  [unwired: 11 in]
      n219 = call "BRig_dataExp_L_freq_l2.vi"() -> ("output_L_freq_l2"=w288:i32)  [unwired: 11 in]
      n220 = call "BRig_dataExp_L_T_l2.vi"() -> ("output_L_T_l2"=w287:i32)  [unwired: 11 in]
      n221 = call "BRig_dataExp_L_Tpeak_l2.vi"() -> ("output_L_Tpeak_l2"=w286:i32)  [unwired: 11 in]
      n222 = call "BRig_dataExp_L_Tshutter_l2.vi"() -> ("output_L_Tshutter_l2"=w285:i32)  [unwired: 11 in]
      n223 = call "BRig_dataExp_L_power_min_l2.vi"() -> ("output_L_power_min_l2"=w284:i32)  [unwired: 11 in]
      n224 = call "BRig_dataExp_L_power_max_l2.vi"() -> ("output_L_power_max_l2"=w283:i32)  [unwired: 11 in]
      n225 = call "BRig_dataExp_L_power_step_l2.vi"() -> ("output_L_power_step_l2"=w282:i32)  [unwired: 11 in]
      n226 = Index Array(array=w371, index #1=w317, index #2=w315, index #3=w316, index #4=w318, index #5=w319, index #6=w320, index #7=w321, index #8=w322, index #9=w323, index #10=w324, index #11=w325, index #12=w326, index #13=w327, index #14=w328, index #15=w329, index #16=w330, index #17=w331, index #18=w332) -> (element #1=w419:u16, element #2=w418:u16, element #3=w417:u16, element #4=w416:u16, element #5=w415:u16, element #6=w414:u16, element #7=w413:u16, element #8=w412:u16, element #9=w411:u16, element #10=w410:u16, element #11=w409:u16, element #12=w408:u16, element #13=w407:u16, element #14=w406:u16, element #15=w405:u16, element #16=w404:u16, element #17=w403:u16, element #18=w402:u16)
      n227 = Index Array(array=w281, index #1=w289, index #2=w288, index #3=w287, index #4=w286, index #5=w285, index #6=w284, index #7=w283, index #8=w282) -> (element #1=w370:u16, element #2=w368:u16, element #3=w367:u16, element #4=w366:u16, element #5=w365:u16, element #6=w364:u16, element #7=w363:u16, element #8=w362:u16)
      n228 = To Double Precision Float(number=w364) -> (double precision float=w361:dbl)
      n229 = To Double Precision Float(number=w363) -> (double precision float=w356:dbl)
      n230 = To Double Precision Float(number=w362) -> (double precision float=w355:dbl)
      n231 = Not Equal To 0?(x=w419) -> (x != 0?=w425:bool)
      n232 = Not Equal To 0?(x=w415) -> (x != 0?=w424:bool)
      n233 = Not Equal To 0?(x=w413) -> (x != 0?=w423:bool)
      n234 = Not Equal To 0?(x=w409) -> (x != 0?=w422:bool)
      n235 = Not Equal To 0?(x=w407) -> (x != 0?=w421:bool)
      n236 = Not Equal To 0?(x=w403) -> (x != 0?=w420:bool)
      n237 = Divide(x=w361, y=w357) -> (x/y=w360:dbl)
      n238 = Divide(x=w356, y=w357) -> (x/y=w359:dbl)
      n239 = Divide(x=w355, y=w357) -> (x/y=w358:dbl)
      n240 = local write "LC_Cue_First_OnOff"(w425) -> ()
      n241 = local write "LC_Cue_First_Block"(w418) -> ()
      n242 = local write "LC_Cue_First_Probability"(w417) -> ()
      n243 = local write "LC_Cue_First_Tdelay"(w416) -> ()
      n244 = local write "LC_Cue_First_delayOpt"(w424) -> ()
      n245 = local write "LC_Cue_First_Count"(w414) -> ()
      n246 = local write "LC_Cue_PreR_OnOff"(w423) -> ()
      n247 = local write "LC_Cue_PreR_Block"(w412) -> ()
      n248 = local write "LC_Cue_PreR_Probability"(w411) -> ()
      n249 = local write "LC_Cue_PreR_Tdelay"(w410) -> ()
      n250 = local write "LC_Cue_PreR_delayOpt"(w422) -> ()
      n251 = local write "LC_Cue_PreR_Count"(w408) -> ()
      n252 = local write "LC_Cue_PostR_OnOff"(w421) -> ()
      n253 = local write "LC_Cue_PostR_Block"(w406) -> ()
      n254 = local write "LC_Cue_PostR_Probability"(w405) -> ()
      n255 = local write "LC_Cue_PostR_Tdelay"(w404) -> ()
      n256 = local write "LC_Cue_PostR_delayOpt"(w420) -> ()
      n257 = local write "LC_Cue_PostR_Count"(w402) -> ()
      n258 = Not Equal To 0?(x=w370) -> (x != 0?=w369:bool)
      n259 = local write "LED_baseline"(w369) -> ()
      n260 = local write "Laser_Freq"(w368) -> ()
      n261 = local write "Laser_T"(w367) -> ()
      n262 = local write "Laser_Tpeak"(w366) -> ()
      n263 = local write "Laser_Tshutter"(w365) -> ()
      n264 = local write "Laser_power_min"(w360) -> ()
      n265 = local write "Laser_power_max"(w359) -> ()
      n266 = local write "Laser_power_step"(w358) -> ()
      n267 = call "BRig_dataLC_ENL_PostR_nRew1_l2.vi"() -> ("output_ENL_PostR_nRew1_l2"=w270:i32)  [unwired: 11 in]
      n268 = call "BRig_dataLC_ENL_PostR_nRew2_l2.vi"() -> ("output_ENL_PostR_nRew2_l2"=w269:i32)  [unwired: 11 in]
      n269 = call "BRig_dataLC_Selection_PostR_nRew1_l2.vi"() -> ("output_Selection_PostR_nRew1_l2"=w266:i32)  [unwired: 11 in]
      n270 = call "BRig_dataLC_Selection_PostR_nRew2_l2.vi"() -> ("output_Selection_PostR_nRew2_l2"=w265:i32)  [unwired: 11 in]
      n271 = call "BRig_dataLC_Cue_PostR_nRew1_l2.vi"() -> ("output_Cue_PostR_nRew1_l2"=w268:i32)  [unwired: 11 in]
      n272 = call "BRig_dataLC_Cue_PostR_nRew2_l2.vi"() -> ("output_Cue_PostR_nRew2_l2"=w267:i32)  [unwired: 11 in]
      n273 = Index Array(array=w281, index #1=w270, index #2=w269, index #3=w268, index #4=w267, index #5=w266, index #6=w265) -> (element #1=w272:u16, element #2=w353:u16, element #3=w352:u16, element #4=w351:u16, element #5=w271:u16, element #6=w354:u16)
      n274 = call "BRig_dataLC_Selection_First_OnOff_l2.vi"() -> ("output_Selection_First_OnOff_l2"=w314:i32)  [unwired: 11 in]
      n275 = call "BRig_dataLC_Selection_First_Block_l2.vi"() -> ("output_Selection_First_Block_l2"=w313:i32)  [unwired: 11 in]
      n276 = call "BRig_dataLC_Selection_First_Prob_l2.vi"() -> ("output_Selection_First_Prob_l2"=w312:i32)  [unwired: 11 in]
      n277 = call "BRig_dataLC_Selection_First_Delay_l2.vi"() -> ("output_Selection_First_Delay_l2"=w311:i32)  [unwired: 11 in]
      n278 = call "BRig_dataLC_Selection_First_Count_l2.vi"() -> ("output_Selection_First_Count_l2"=w310:i32)  [unwired: 11 in]
      n279 = call "BRig_dataLC_Selection_PreR_OnOff_l2.vi"() -> ("output_Selection_PreR_OnOff_l2"=w309:i32)  [unwired: 11 in]
      n280 = call "BRig_dataLC_Selection_PreR_Block_l2.vi"() -> ("output_Selection_PreR_Block_l2"=w308:i32)  [unwired: 11 in]
      n281 = call "BRig_dataLC_Selection_PreR_Prob_l2.vi"() -> ("output_Selection_PreR_Prob_l2"=w307:i32)  [unwired: 11 in]
      n282 = call "BRig_dataLC_Selection_PreR_Delay_l2.vi"() -> ("output_Selection_PreR_Delay_l2"=w306:i32)  [unwired: 11 in]
      n283 = call "BRig_dataLC_Selection_PreR_Count_l2.vi"() -> ("output_Selection_PreR_Count_l2"=w305:i32)  [unwired: 11 in]
      n284 = call "BRig_dataLC_Selection_PostR_OnOff_l2.vi"() -> ("output_Selection_PostR_OnOff_l2"=w304:i32)  [unwired: 11 in]
      n285 = call "BRig_dataLC_Selection_PostR_Block_l2.vi"() -> ("output_Selection_PostR_Block_l2"=w303:i32)  [unwired: 11 in]
      n286 = call "BRig_dataLC_Selection_PostR_Prob_l2.vi"() -> ("output_Selection_PostR_Prob_l2"=w302:i32)  [unwired: 11 in]
      n287 = call "BRig_dataLC_Selection_PostR_Delay_l2.vi"() -> ("output_Selection_PostR_Delay_l2"=w301:i32)  [unwired: 11 in]
      n288 = call "BRig_dataLC_Selection_PostR_Count_l2.vi"() -> ("output_Selection_PostR_Count_l2"=w300:i32)  [unwired: 11 in]
      n289 = call "BRig_dataLC_Reward_OnOff_l2.vi"() -> ("output_Reward_OnOff_l2"=w290:i32)  [unwired: 11 in]
      n290 = call "BRig_dataLC_Reward_Block_l2.vi"() -> ("output_Reward_Block_l2"=w291:i32)  [unwired: 11 in]
      n291 = call "BRig_dataLC_Reward_Trial_l2.vi"() -> ("output_Reward_Trial_l2"=w292:i32)  [unwired: 11 in]
      n292 = call "BRig_dataLC_Reward_Prob_l2.vi"() -> ("output_Reward_Prob_l2"=w293:i32)  [unwired: 11 in]
      n293 = call "BRig_dataLC_Reward_Delay_l2.vi"() -> ("output_Reward_Delay_l2"=w294:i32)  [unwired: 11 in]
      n294 = call "BRig_dataLC_Wrong_OnOff_l2.vi"() -> ("output_Wrong_OnOff_l2"=w295:i32)  [unwired: 11 in]
      n295 = call "BRig_dataLC_Wrong_Block_l2.vi"() -> ("output_Wrong_Block_l2"=w296:i32)  [unwired: 11 in]
      n296 = call "BRig_dataLC_Wrong_Trial_l2.vi"() -> ("output_Wrong_Trial_l2"=w297:i32)  [unwired: 11 in]
      n297 = call "BRig_dataLC_Wrong_Prob_l2.vi"() -> ("output_Wrong_Prob_l2"=w298:i32)  [unwired: 11 in]
      n298 = call "BRig_dataLC_Wrong_Delay_l2.vi"() -> ("output_Wrong_Delay_l2"=w299:i32)  [unwired: 11 in]
      n299 = Index Array(array=w371, index #1=w290, index #2=w291, index #3=w292, index #4=w293, index #5=w294, index #6=w295, index #7=w296, index #8=w297, index #9=w298, index #10=w299) -> (element #1=w381:u16, element #2=w380:u16, element #3=w379:u16, element #4=w378:u16, element #5=w377:u16, element #6=w376:u16, element #7=w375:u16, element #8=w374:u16, element #9=w373:u16, element #10=w372:u16)
      n300 = Index Array(array=w371, index #1=w314, index #2=w313, index #3=w312, index #4=w311, index #5=w310, index #6=w309, index #7=w308, index #8=w307, index #9=w306, index #10=w305, index #11=w304, index #12=w303, index #13=w302, index #14=w301, index #15=w300) -> (element #1=w398:u16, element #2=w397:u16, element #3=w396:u16, element #4=w395:u16, element #5=w394:u16, element #6=w393:u16, element #7=w392:u16, element #8=w391:u16, element #9=w390:u16, element #10=w389:u16, element #11=w388:u16, element #12=w387:u16, element #13=w386:u16, element #14=w385:u16, element #15=w384:u16)
      n301 = local write "LC_ENL_nRew2"(w353) -> ()
      n302 = local write "LC_ENL_nRew1"(w272) -> ()
      n303 = local write "LC_Cue_nRew2"(w351) -> ()
      n304 = local write "LC_Sel_nRew2"(w354) -> ()
      n305 = local write "LC_Sel_nRew1"(w271) -> ()
      n306 = local write "LC_Cue_nRew1"(w352) -> ()
      n307 = Not Equal To 0?(x=w381) -> (x != 0?=w383:bool)
      n308 = Not Equal To 0?(x=w376) -> (x != 0?=w382:bool)
      n309 = Not Equal To 0?(x=w398) -> (x != 0?=w401:bool)
      n310 = Not Equal To 0?(x=w393) -> (x != 0?=w400:bool)
      n311 = Not Equal To 0?(x=w388) -> (x != 0?=w399:bool)
      n312 = local write "LC_Reward_OnOff"(w383) -> ()
      n313 = local write "LC_Reward_Block"(w380) -> ()
      n314 = local write "LC_Reward_Trial"(w379) -> ()
      n315 = local write "LC_Reward_Probability"(w378) -> ()
      n316 = local write "LC_Reward_Tdelay"(w377) -> ()
      n317 = local write "LC_Wrong_OnOff"(w382) -> ()
      n318 = local write "LC_Wrong_Block"(w375) -> ()
      n319 = local write "LC_Wrong_Trial"(w374) -> ()
      n320 = local write "LC_Wrong_Probability"(w373) -> ()
      n321 = local write "LC_Wrong_Tdelay"(w372) -> ()
      n322 = local write "LC_Sel_First_OnOff"(w401) -> ()
      n323 = local write "LC_Sel_First_Block"(w397) -> ()
      n324 = local write "LC_Sel_First_Probability"(w396) -> ()
      n325 = local write "LC_Sel_First_Tdelay"(w395) -> ()
      n326 = local write "LC_Sel_First_Count"(w394) -> ()
      n327 = local write "LC_Sel_PreR_OnOff"(w400) -> ()
      n328 = local write "LC_Sel_PreR_Block"(w392) -> ()
      n329 = local write "LC_Sel_PreR_Probability"(w391) -> ()
      n330 = local write "LC_Sel_PreR_Tdelay"(w390) -> ()
      n331 = local write "LC_Sel_PreR_Count"(w389) -> ()
      n332 = local write "LC_Sel_PostR_OnOff"(w399) -> ()
      n333 = local write "LC_Sel_PostR_Block"(w387) -> ()
      n334 = local write "LC_Sel_PostR_Probability"(w386) -> ()
      n335 = local write "LC_Sel_PostR_Tdelay"(w385) -> ()
      n336 = local write "LC_Sel_PostR_Count"(w384) -> ()
    }
  }
  "output_dataLC" <- w4
  "output_dataExp" <- w1
